vi "Select Control Type.vi"(8 "error in (no error)":errorcluster, 10 "Control Type":string, 11 "Editor in":refnum<class "Editor.lvclass">) -> (0 "error out":errorcluster, 3 "Editor out":refnum<class "Editor.lvclass">)   [LabVIEW 2020, in "VolatusGUIEditor.lvlib" / "Editor.lvclass"]
uses:
  Editor.lvclass
  Editor.lvclass/Editor.ctl
  Control List/Control List.lvclass
  VolatusGUIEditor.lvlib
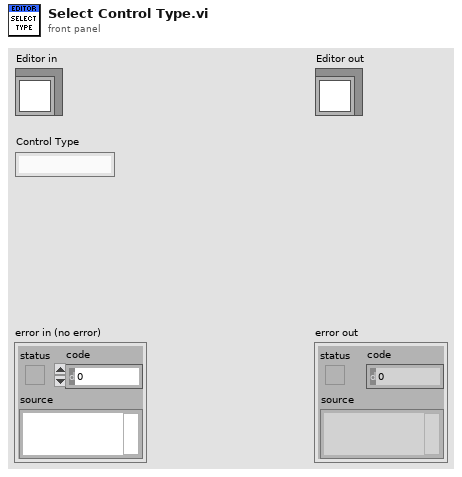
[diagram p1: front panel]
types:
  T1 = typedef "VolatusGUIEditor.lvlib/Control Info.ctl" = cluster{"Description":string, "Hierarchy":string[], "Image":T2}
  T2 = typedef "imagedata.ctl" = cluster{"image type":i32, "image depth":i32, "image":u8[], "mask":u8[], "colors":u32[], "Rectangle":cluster{"left":i16, "top":i16, "right":i16, "bottom":i16}}
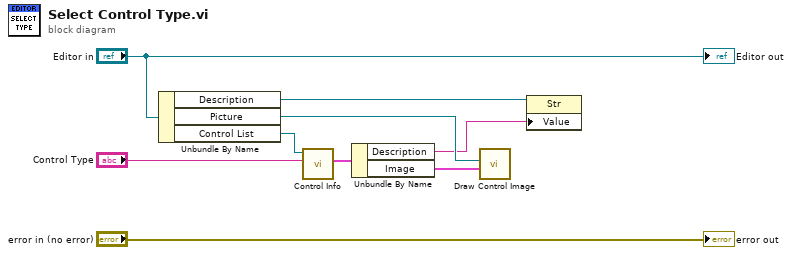
[diagram p0: block diagram]
diagram:
  n1 = Unbundle By Name("Editor in") -> ("Description"=w2:refnum<vi>, "Picture"=w3:refnum<vi>, "Control List"=w7:refnum<class "Control List.lvclass">)
  n2 = call "Control Info.vi"("Control Type"="Control Type", "Control List in"=w7) -> ("Control Info"=w5:T1)  [unwired: 7 in, 2 out]
  n3 = Unbundle By Name(w5) -> ("Description"=w1:string, "Image"=w4:T2)
  n4 = call "Draw Control Image.vi"("Image"=w4, "Picture Ref"=w3) -> ()  [unwired: 10 in]
  n5 = property class="Str"(reference=w2, "Value"=w1) -> ()  [unwired: 1 in, 2 out]
  "error out" <- "error in (no error)"
  "Editor out" <- "Editor in"
